vi "Init Config.vi"(8 "error in (no error)":errorcluster, 11 "App in":refnum<class "App.lvclass">) -> (0 "error out":errorcluster, 3 "App out":refnum<class "App.lvclass">)   [LabVIEW 2020, in "PicoG-App.lvlib" / "App.lvclass"]
uses:
  App.lvclass
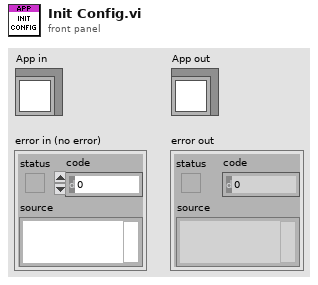
[diagram p1: front panel]
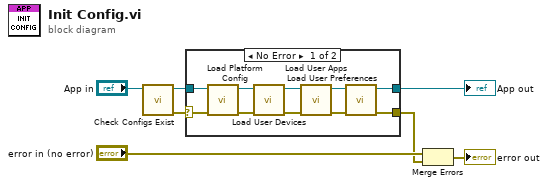
[diagram p0: block diagram]
diagram:
  n1 = call "Check Configs Exist.vi"("App in"="App in") -> ("error out"=w5:errorcluster, "App out"=w3:refnum<class "App.lvclass">)  [unwired: 9 in]
  n2 = case shown="No Error" w5 {
    selector: w5 -> [w12 w19]
    tunnel: [w9 w19] -> w1
    tunnel: w3 -> [w13 w18]
    tunnel: [w8 w18] -> w2
    frame No Error {
      n3 = call "Load Platform Config.vi"("error in (no error)"=w12, "App in"=w13) -> ("error out"=w15:errorcluster, "App out"=w14:refnum<class "App.lvclass">)  [unwired: 8 in]
      n4 = call "Load User Devices.vi"("error in (no error)"=w15, "App in"=w14) -> ("error out"=w17:errorcluster, "App out"=w16:refnum<class "App.lvclass">)  [unwired: 8 in]
      n5 = call "Load User Apps.vi"("error in (no error)"=w17, "App in"=w16) -> ("error out"=w10:errorcluster, "App out"=w11:refnum<class "App.lvclass">)  [unwired: 8 in]
      n6 = call "Load User Preferences.vi"("error in (no error)"=w10, "App in"=w11) -> ("error out"=w9:errorcluster, "App out"=w8:refnum<class "App.lvclass">)  [unwired: 8 in]
    }
    frame Error {
    }
  }
  "App out" <- w2
  n7 = Merge Errors("error in (no error)", w1) -> (→"error out":errorcluster)
